vi "Add Dependency Shape.vi"(8 "error in (no error)":errorcluster, 9 "Dependency Shape":refnum<data-value>, 11 "Shape Ref in":refnum<data-value>) -> (0 "error out":errorcluster, 3 "Shape Ref Out":refnum<data-value>)   [LabVIEW 2017, in "LV Image Editor Framework.lvlib" / "Shape.lvclass"]
uses:
  Shape.lvclass
  Shape.lvclass/Shape.ctl
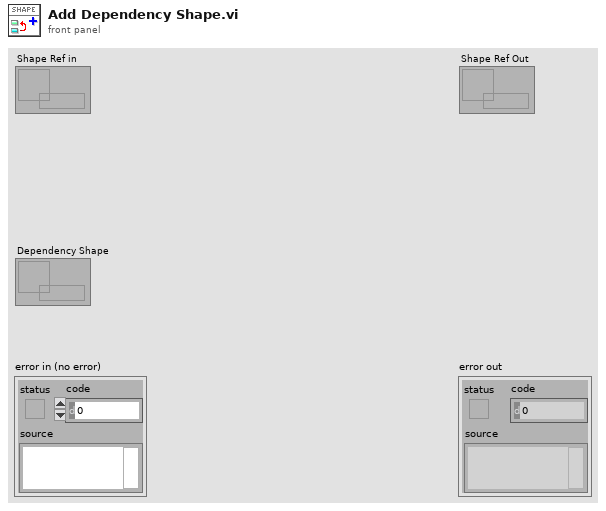
[diagram p1: front panel]
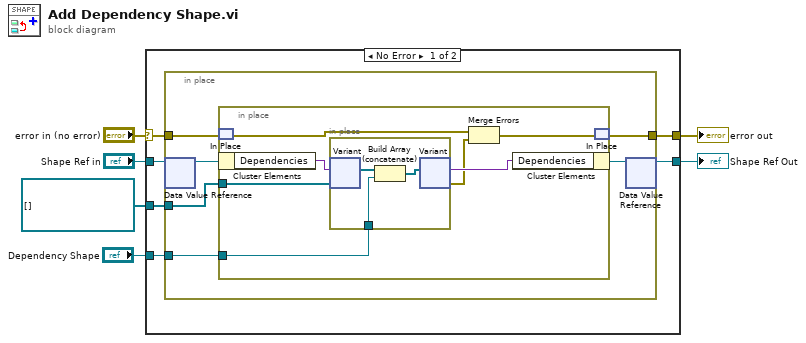
[diagram p0: block diagram]
diagram:
  n1 = case shown="No Error" "error in (no error)" {
    selector: "error in (no error)" -> [w11 w30]
    tunnel: [w10 w30] -> w5
    tunnel: "Dependency Shape" -> [w12 _]
    tunnel: "Shape Ref in" -> [w9 w29]
    tunnel: [w8 w29] -> w2
    tunnel: refnum<data-value>[] [] ("Dependency Shape") -> [w7 _]
    frame No Error {
      n2 = in-place {
        in-place-border: w12 -> [w18]
        in-place-border: w11 -> [w17]
        in-place-border: [w16] -> w10
        in-place-border: w7 -> [w13]
        n3 = in-place-dvr #1(w9) -> (w15:refnum<class "Shape.lvclass">)  [unwired: 1 out]
        n4 = in-place {
          in-place-border: w18 -> [w23]
          in-place-border: w13 -> [w24]
          n5 = in-place-match #2(w17) -> (w19:errorcluster)
          n6 = in-place-cluster #3(w15) -> ("Dependencies"=w25:variant)
          n7 = in-place {
            in-place-border: w23 -> [w27]
            n8 = in-place-variant #4(w25, w24) -> (w28:refnum<data-value>[])  [unwired: 1 out]
            n9 = Build Array (concatenate)(w28, w27) -> (w26:refnum<data-value>[])
            n10 = in-place-variant #4(w26) -> (w22:variant, w20:errorcluster)
          }
          n11 = Merge Errors(w19, w20) -> (w21:errorcluster)
          n12 = in-place-cluster #3("Dependencies"=w22) -> (w14:refnum<class "Shape.lvclass">)
          n13 = in-place-match #2(w21) -> (w16:errorcluster)
        }
        n14 = in-place-dvr #1(w14) -> (w8:refnum<data-value>)  [unwired: 1 out]
      }
    }
    frame Error {
    }
  }
  "error out" <- w5
  "Shape Ref Out" <- w2
